vi "Job selector.vi"() -> ()   [LabVIEW 2010]
uses:
  GUI/Job setup/Job and site cluster.ctl
  emi cndiates/List of all contrys(combo box).ctl
  GUI/Job setup/Tool registration ID.ctl
  GUI/Job setup/Operators display clustor.ctl
panel:
  in  "Open project":bool
  in  "Ring":u16(ring)
  in  "New project":bool
  in  "Operators":T1
  out "Tool":T2
  out "Job & Site":T3
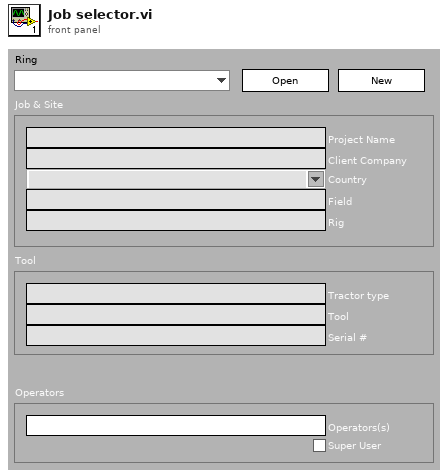
[diagram p1: front panel]
types:
  T1 = typedef "Operators display clustor.ctl" = cluster{"Operators(s)":string, "Super User":bool}
  T2 = typedef "Tool registration ID.ctl" = cluster{"Tractor type":string, "Tool":string, "Serial #":string}
  T3 = typedef "Job and site cluster.ctl" = cluster{"Project Name":string, "Client Company":string, "Field":string, "Rig":string, "Country":T4}
  T4 = typedef "List of all contrys(combo box).ctl" = string
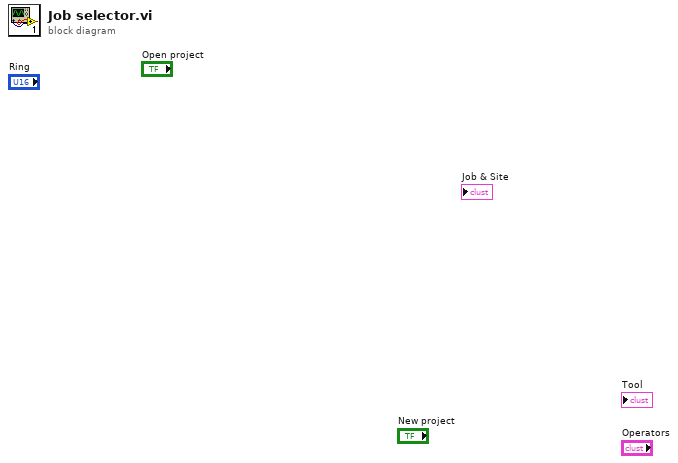
[diagram p0: block diagram]
diagram:
